vi "getOutputGain.vi"(8 "error in (no error)":errorcluster, 11 "Instrument.LockinAPI in":refnum<class "Instrument.LockinAPI.lvclass">) -> (0 "error out":errorcluster, 2 "OutputGain":dbl[](array[numeric]), 3 "Instrument.LockinAPI out":refnum<class "Instrument.LockinAPI.lvclass">)   [LabVIEW 2019, in "Instrument.LockinAPI.lvclass"]
doc: "API to get the AI waveforms.\n\nIf address=\"\", this API reads from localhost\nIf address is remote lockin, you need to add this computer to allowed whitelist on the lockin computer you are trying to access."
uses:
  Instrument.LockinAPI.lvclass
  C:/Users/patrick/Documents/GitHub/Instrument-Framework/lvsrc/Instrument/Instrument.lvclass
  Typedefs/API/LockinAPI.Commands--Enum.ctl
  dfa3ef30-9e3a-43bb-a6e8-fdc027893c94.vi
  dfa3ef30-9e3a-43bb-a6e8-fdc027893c94.vi/2163da24-5c82-49a0-ac1f-a7aa94482ef6.vi
  dfa3ef30-9e3a-43bb-a6e8-fdc027893c94.vi/2163da24-5c82-49a0-ac1f-a7aa94482ef6.vi/6ddc0ee9-da63-42f5-b5cd-1cfeb561a303.vi
  dfa3ef30-9e3a-43bb-a6e8-fdc027893c94.vi/2163da24-5c82-49a0-ac1f-a7aa94482ef6.vi/ed4d24ca-279d-497a-84cf-6a54bd5046ac.vi
  dfa3ef30-9e3a-43bb-a6e8-fdc027893c94.vi/2163da24-5c82-49a0-ac1f-a7aa94482ef6.vi/c6a54e7a-b7b6-4897-b0c2-bbd824f2b017.vi
  <vilib>/JDP Science/JSONtext/Make JSON Array.vi
  dfa3ef30-9e3a-43bb-a6e8-fdc027893c94.vi/2163da24-5c82-49a0-ac1f-a7aa94482ef6.vi/ed4d24ca-279d-497a-84cf-6a54bd5046ac.vi/5111ca92-f112-4406-92a4-57786dd0bc15.vi
  dfa3ef30-9e3a-43bb-a6e8-fdc027893c94.vi/2163da24-5c82-49a0-ac1f-a7aa94482ef6.vi/c6a54e7a-b7b6-4897-b0c2-bbd824f2b017.vi/29457455-f266-4d1b-bcad-e7cca947d7a5.vi
  dfa3ef30-9e3a-43bb-a6e8-fdc027893c94.vi/2163da24-5c82-49a0-ac1f-a7aa94482ef6.vi/c6a54e7a-b7b6-4897-b0c2-bbd824f2b017.vi/907e1597-b8c5-40d5-8dfd-81a8d7c44947.vi
  Instrument/API/Enum to String.vi
  Instrument/Private/Get RC Connection Status.vi
  <vilib>/JDP Science/JSONtext/Variant to JSON Text.vi
  <vilib>/JDP Science/JSONtext/support/Format JSON Array Text.vi
  Instrument/API/Send and Receive.vi
  <vilib>/JDP Science/JSONtext/JSON text to Variant.vi
  <vilib>/Utility/Data Type/Get Type Information.vi
  <vilib>/JDP Science/JSONtext/LVClass Serializer/JSONtext LVClass Serializer.lvclass
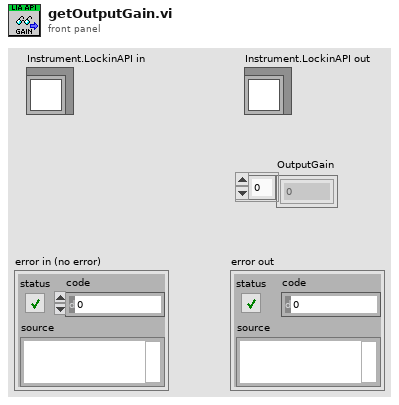
[diagram p1: front panel]
types:
  T1 = typedef "Instrument.LockinAPI.lvclass/LockinAPI.Commands--Enum.ctl" = enum16{"setAI", "setAO", "setAO_Amplitude", "setAO_DC", "setAO_Frequency", "setAO_Phase", "setAO_Function", "setAO_I+", "setREF", "setREF_Frequency", "setREF_Phase", "setREF_TC", "setREF_Roll-Off", "setDAQ", "setSampling", "setOffset", "setState", "getState", "getAO", "getAI", "getResults", "getSampling", "getAOconfig", "getREFconfig", "setInputGain", "setOutputGain", "getInputGain", "getOutputGain", "setSamplingMode", "getSamplingMode", "setSweep", "setSweepTime", "setSweepTable", "getStatus", "getSweepResults", "getSweepWaveforms", "startSweep", "stopSweep", "setAUX", "getAUX"}
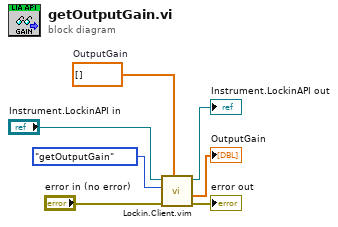
[diagram p0: block diagram]
diagram:
  w2 = dbl[] []  # OutputGain
  n1 = call "Lockin.Client.vim"("Data Out type"=w2, "error in (no error)"="error in (no error)", "Command"=LockinAPI.Commands--Enum."getOutputGain", "Instrument.LockinAPI in"="Instrument.LockinAPI in") -> ("error out"=→"error out":errorcluster, "Data out"=→"OutputGain":dbl[], "Instrument.LockinAPI out"=→"Instrument.LockinAPI out":refnum<class "Instrument.LockinAPI.lvclass">)  [unwired: 5 in]
